vi "SRX_Read_ Sensor Values.vi"(8 "Error":errorcluster, 9 "PidLoopIdx":u32, 11 "PhoenixMotorControlDevRef":T1) -> (0 "Error Out":errorcluster, 2 "Encoder Values Out":T6, 3 "PhoenixMotorControlDevRef Out":T1)   [LabVIEW 2023]
uses:
  Shared Code/TypeDefs/Cluster_FX Sensor Values.ctl
  <vilib>/Rock Robotics/WPI/MotorControl/WPI_MotorControlDeviceRef.ctl
  <vilib>/Rock Robotics/WPI/MotorControl/WPI_MotorControlType.ctl
  <vilib>/Rock Robotics/SystemInterfaces/DIO/FPGA_DIOPWMChannel.ctl
  <vilib>/Rock Robotics/WPI/PWM/WPI_PWMDeadband.ctl
  <vilib>/Rock Robotics/SystemInterfaces/DIO/FPGA_DIOChannel.ctl
  <vilib>/Rock Robotics/WPI/ThirdParty/Phoenix-LabVIEW/Motor Controller/Get/CTRE_Phoenix_MotorController_GetSelectedSensorData.vi
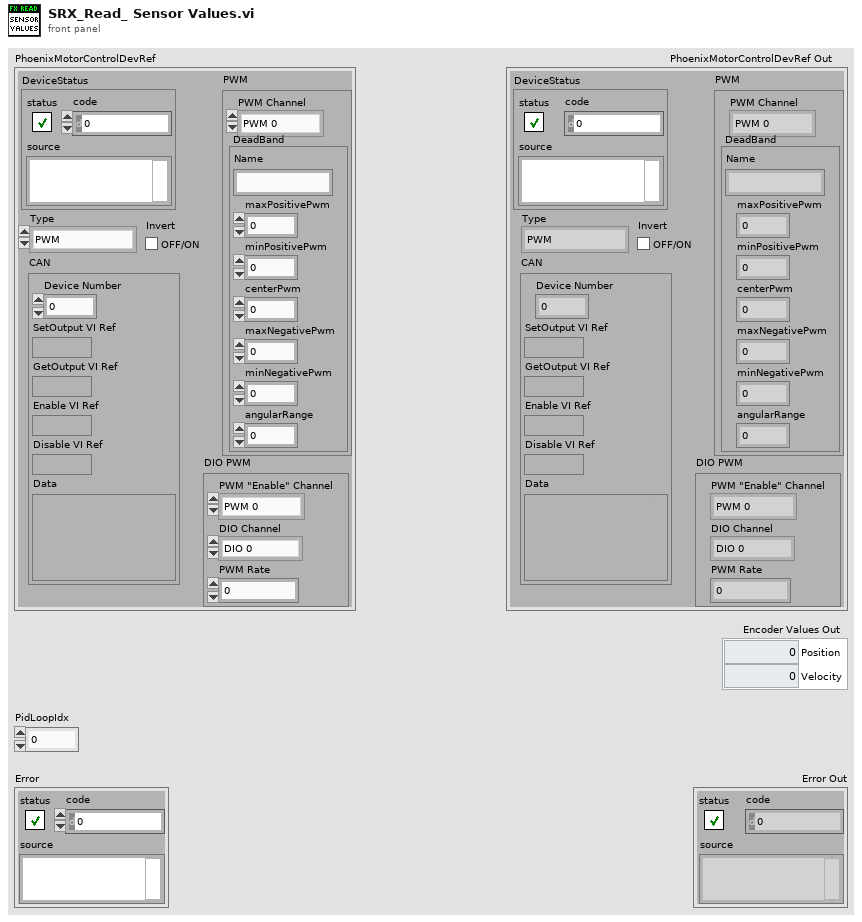
[diagram p1: front panel]
types:
  T1 = typedef "WPI_MotorControlDeviceRef.ctl" = cluster{"DeviceStatus":errorcluster, "Type":T2, "PWM":cluster{"PWM Channel":T3, "DeadBand":T4}, "CAN":cluster{"Device Number":u8, "SetOutput VI Ref":variant, "GetOutput VI Ref":variant, "Enable VI Ref":variant, "Disable VI Ref":variant, "Data":variant}, "Invert":bool, "DIO PWM":cluster{"PWM \"Enable\" Channel":T3, "DIOChannel":T5, "PWM Rate":dbl}}
  T2 = typedef "WPI_MotorControlType.ctl" = enum16{"PWM", "CAN", "DIO PWM"}
  T3 = typedef "FPGA_DIOPWMChannel.ctl" = enum8{"PWM 0", "PWM 1", "PWM 2", "PWM 3", "PWM 4", "PWM 5", "PWM 6", "PWM 7", "PWM 8", "PWM 9", "PWM MXP 0", "PWM MXP 1", "PWM MXP 2", "PWM MXP 3", "PWM MXP 4", "PWM MXP 5", "PWM MXP 6", "PWM MXP 7", "PWM MXP 8", "PWM MXP 9", "Invalid"}
  T4 = typedef "WPI_PWMDeadband.ctl" = cluster{"Name":string, "maxPositivePwm":i32, "minPositivePwm":i32, "centerPwm":i32, "maxNegativePwm":i32, "minNegativePwm":i32, "angularRange":u16}
  T5 = typedef "FPGA_DIOChannel.ctl" = enum8{"DIO 0", "DIO 1", "DIO 2", "DIO 3", "DIO 4", "DIO 5", "DIO 6", "DIO 7", "DIO 8", "DIO 9", "DIO MXP 0", "DIO MXP 1", "DIO MXP 2", "DIO MXP 3", "DIO MXP 4", "DIO MXP 5", "DIO MXP 6", "DIO MXP 7", "DIO MXP 8", "DIO MXP 9", "DIO MXP 10", "DIO MXP 11", "DIO MXP 12", "DIO MXP 13", "DIO MXP 14", "DIO MXP 15", "SPI Port CS1", "SPI Port CS2", "SPI Port CS3", "SPI Port MISO", "SPI Port MOSI", "Invalid"}
  T6 = typedef "Cluster_FX Sensor Values.ctl" = cluster{"Position":i32, "Velocity":i32}
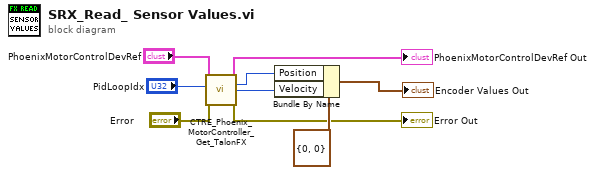
[diagram p0: block diagram]
diagram:
  n1 = call-poly <vilib>:"CTRE_Phoenix_MotorController_Get_TalonFX.vi"("PhoenixMotorControlDevRef"="PhoenixMotorControlDevRef", "pidLoopIdx"="PidLoopIdx", "error in"="Error") -> ("PhoenixMotorControlDevRef"=→"PhoenixMotorControlDevRef Out":T1, "Position (Raw Sensor Units)"=w3:i32, "Velocity (Raw Sensor Units per 100 ms)"=w2:i32, "error out"=→"Error Out":errorcluster)  [unwired: 9 in]
  n2 = Bundle By Name(cluster=T6 {"Position"=0, "Velocity"=0} ("Voltage Data"), "Position"=w3, "Velocity"=w2) -> (→"Encoder Values Out":T6)
